vi "SQL写入 - NG.vi"(0 "WorkNumber":string, 5 "ProductNumber":string, 7 "TestMessage":string, 9 "ProssureType":string, 11 "error in (no error)":errorcluster caption="错误输入（无错误）") -> (4 "ADODB._Connection Out":refnum<k7>, 15 "error out":errorcluster caption="错误输出")   [LabVIEW 2017]
panel:
  in  "Barcode":string
  out "连接的字符串":string
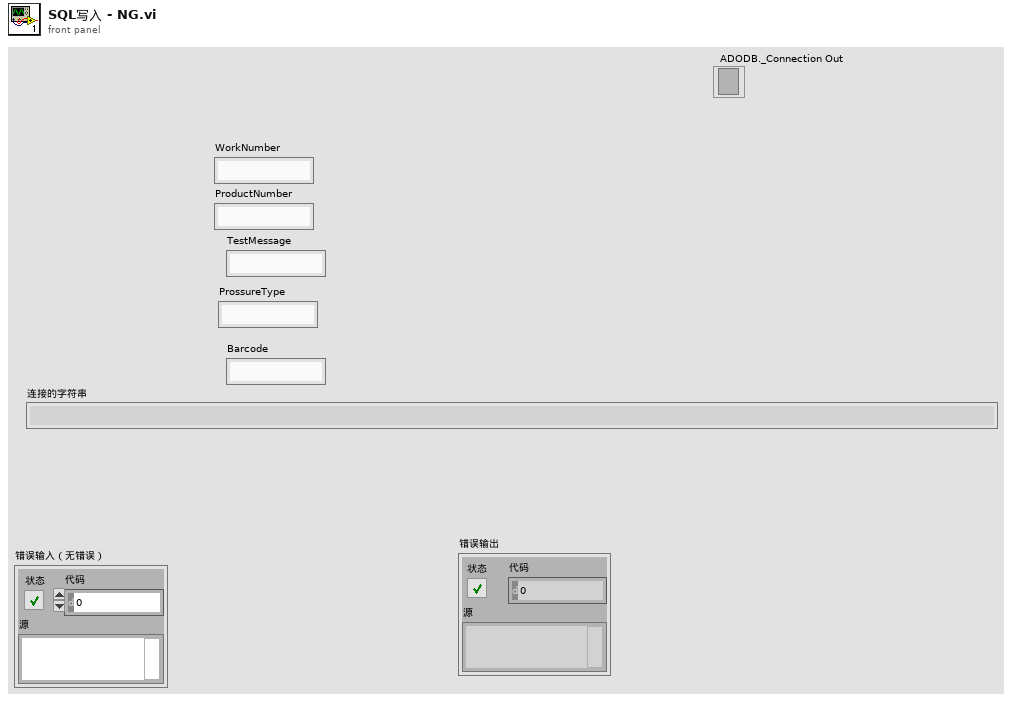
[diagram p1: front panel]
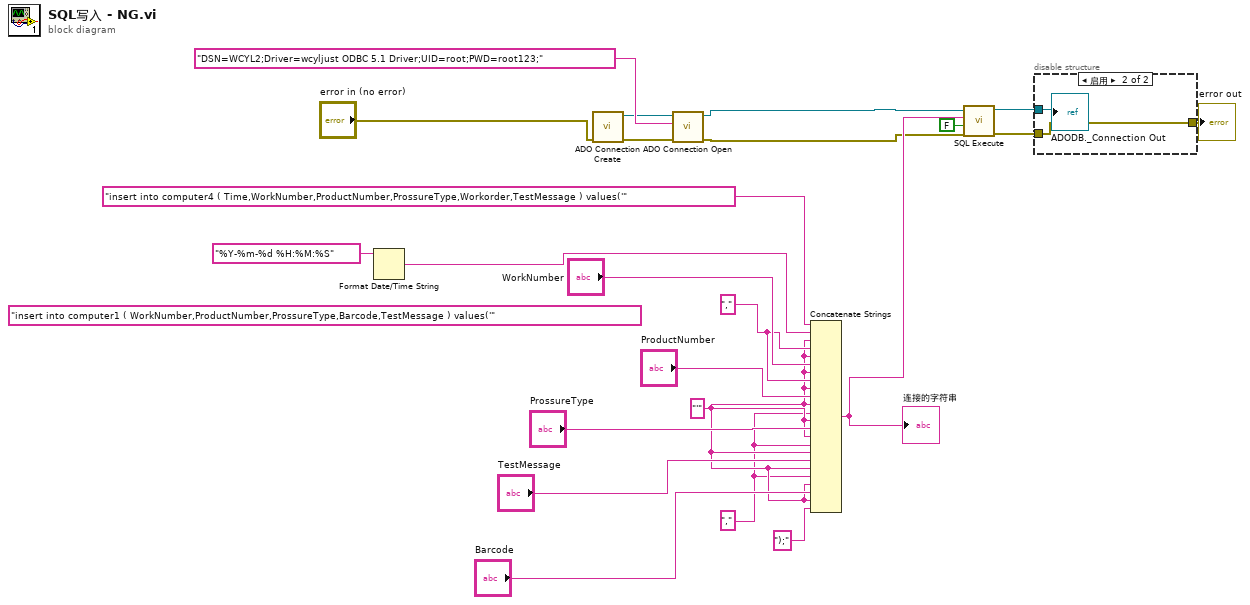
[diagram p0: block diagram]
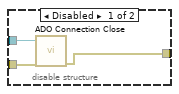
[diagram p2: hidden frame]
diagram:
  (unwired) "insert into computer1 ( WorkNumber,ProductNumber,ProssureType,Barcode,TestMessage ) values('" ("Command Text")
  w10 = "'" ("字符串")
  w1 = "," ("字符串")
  w12 = "," ("字符串")
  n1 = Format Date/Time String(time format string (%c)="%Y-%m-%d %H:%M:%S" ("时间格式字符串(%c)")) -> (date/time string=w13:string)  [unwired: 2 in]
  n2 = call <userlib>:"ADO Connection Create.vi"("error in (no error)"="error in (no error)") -> ("error out"=w8:errorcluster, "ADODB._Connection Out"=w9:refnum<k7>)  [unwired: 9 in]
  n3 = call <userlib>:"ADO Connection Open.vi"("error in (no error)"=w8, "ConnectionString"="DSN=WCYL2;Driver=wcyljust ODBC 5.1 Driver;UID=root;PWD=root123;", "ADODB._Connection In"=w9) -> ("error out"=w3:errorcluster, "ADODB._Connection Out"=w4:refnum<k7>)  [unwired: 7 in]
  n4 = Concatenate Strings("insert into computer4 ( Time,WorkNumber,ProductNumber,ProssureType,Workorder,TestMessage ) values('" ("Command Text"), w13, w10, w12, w10, "WorkNumber", w10, w12, w10, "ProductNumber", w10, w1, w10, "ProssureType", w10, w1, w10, "TestMessage", w10, w1, w10, "Barcode", w10, ");" ("字符串")) -> (w18:string)
  "连接的字符串" <- w18
  n5 = call <userlib>:"SQL Execute.vi"("error in (no error)"=w3, "Return Data (T)"=FALSE, "Command Text"=w18, "ADODB._Connection In"=w4) -> ("error out"=w6:errorcluster, "ADODB._Connection Out"=w7:refnum<k7>)  [unwired: 4 in, 2 out]
  n6 = disable-structure shown="启用" {
    disable-tunnel: [w26 w28] -> w16
    disable-tunnel: w7 -> [w25 w27]
    disable-tunnel: w6 -> [w24 w28]
    frame Disabled {
      n7 = call <userlib>:"ADO Connection Close.vi"("error in (no error)"=w24, "ADODB._Connection In"=w25) -> ("error out"=w26:errorcluster)  [unwired: 8 in, 1 out]
    }
    frame Enabled {
      "ADODB._Connection Out" <- w27
    }
  }
  "error out" <- w16
